vi "CAN_Init - 2013.vi"(0 "设备类型":u32(ring)=4 items=["PCI5121"=1, "PCI9810"=2, "USBCAN1"=3, "USBCAN2"=4, "PCI9820"=5, "CAN232"=6, "PCI5110"=7, "CANLite(mini)"=8, "ISA9620"=9, "ISA5420"=10, "PC104CAN"=11, "CANET"=17, "DNP9810"=13, "USBCAN-E-U"=20, "USBCAN-2E-U"=21], 1 "设备索引":u32(ring) items=["0", "1", "2", "3", "4", "5", "6", "7", "8", "9", "10", "11", "12", "13", "14", "15", ""], 2 "波特率":enum16{"250Kbps", "500Kbps"}(ring)=enum."500Kbps", 3 "CAN路数":u32(ring) items=["0", "1"], 4 "操作类型":enum16{"初始化CAN", "关闭CAN"}(ring), 5 "error in (no error)":errorcluster caption="错误输入（无错误）", 6 "滤波方式":u8(ring)=1 items=["Dual Filter", "Single Filter"], 7 "Accept Code":u32 format="%08x", 8 "IP":string, 9 "port":u32, 10 "工作方式":u8(ring) items=["Normal", "Listen Only"], 11 "Mask Code":u32=4294967295 format="%08x", 12 "PC端-协议类型":enum16{"TCP服务器Server", "TCP客户端Client"}(ring)) -> (14 "CAN 操作结果":bool=TRUE, 19 "error out":errorcluster caption="错误输出")   [LabVIEW 2013]
uses:
  data/ControlCAN.dll
panel:
  in  "VCI_INIT_CONFIG":T1={"AccCode"=0, "AccMask"=4294967295, "Reserved"=0, "Filter"=0, "Timing0"=191, "Timing1"=255, "Mode"=0}
  in  "DeviceType 5":u16(ring)=1 items=["PCI5121"=1, "PCI9810"=2, "USBCAN1"=3, "USBCAN2"=4, "PCI9820"=5, "CAN232"=6, "PCI5110"=7, "CANLite(mini)"=8, "ISA9620"=9, "ISA5420"=10, "PC104CAN"=11, "CANETE"=12, "DNP9810"=13]
  in  "CAN Channel 3":u16(ring) items=["0", "1"]
  in  "DeviceType 4":u16(ring)=1 items=["PCI5121"=1, "PCI9810"=2, "USBCAN1"=3, "USBCAN2"=4, "PCI9820"=5, "CAN232"=6, "PCI5110"=7, "CANLite(mini)"=8, "ISA9620"=9, "ISA5420"=10, "PC104CAN"=11, "CANETE"=12, "DNP9810"=13]
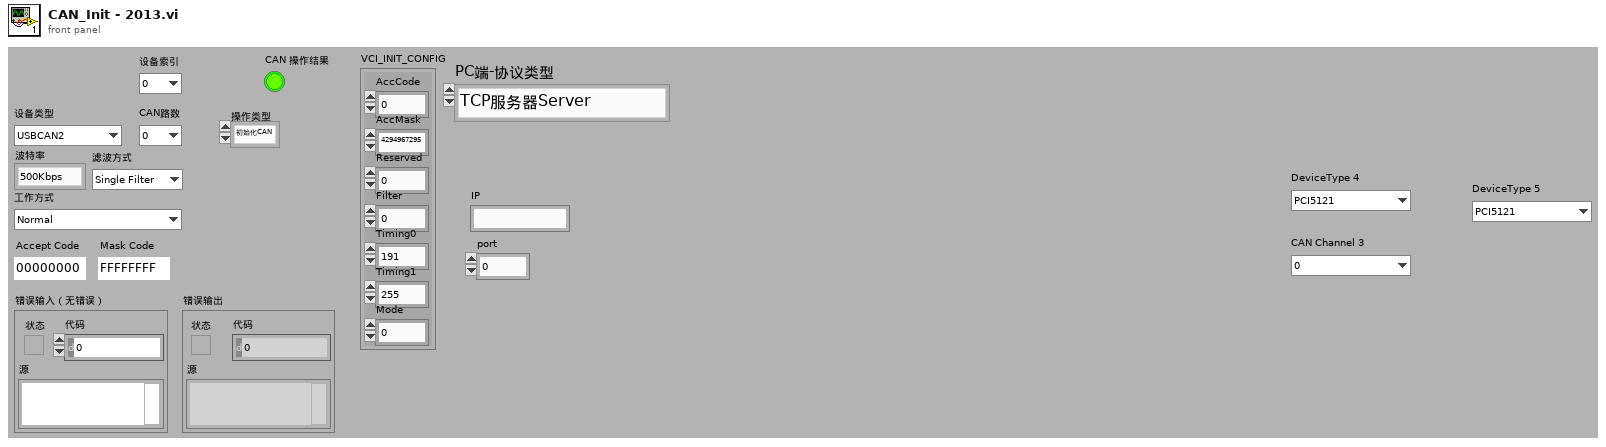
[diagram p1: front panel]
types:
  T1 = cluster{"AccCode":u32, "AccMask":u32, "Reserved":u32, "Filter":u8, "Timing0":u8, "Timing1":u8, "Mode":u8}
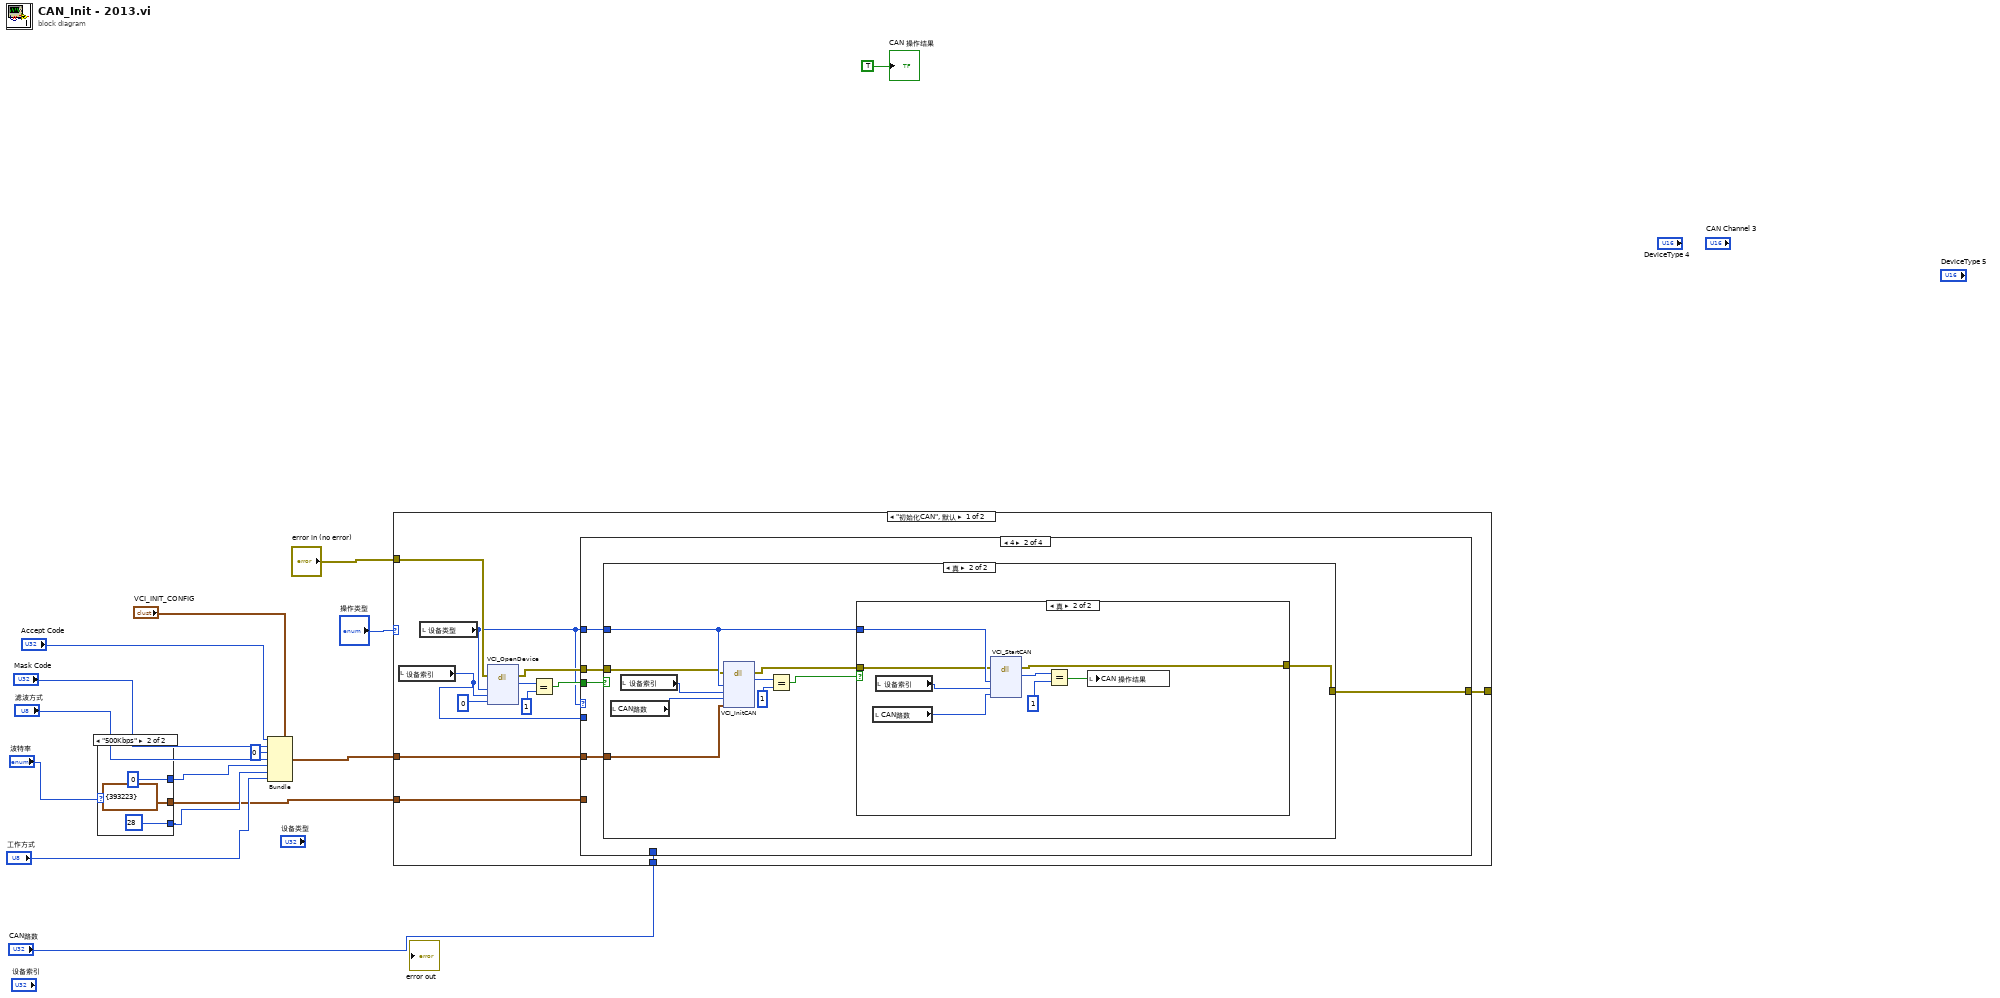
[diagram p0: block diagram]
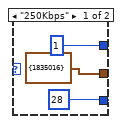
[diagram p2: hidden frame]
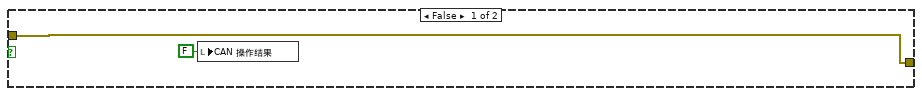
[diagram p4: hidden frame]
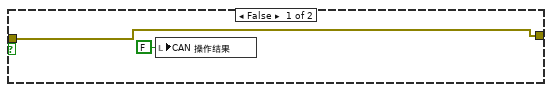
[diagram p5: hidden frame]
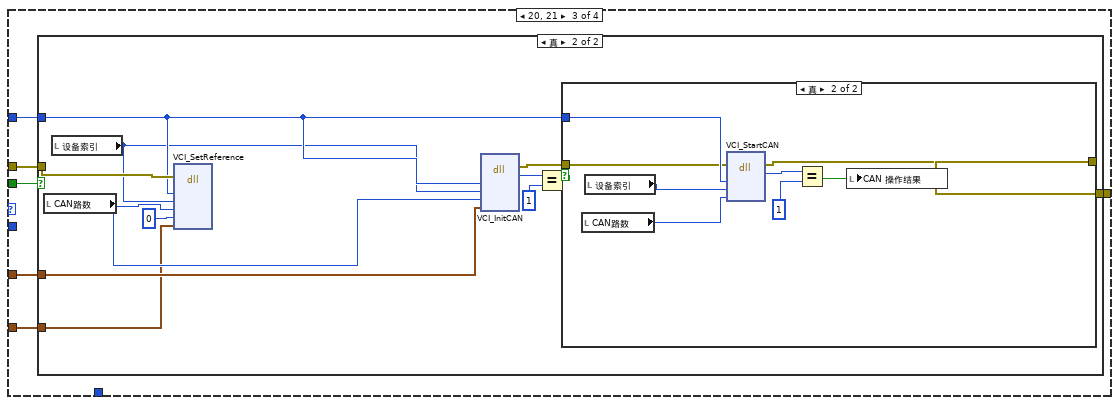
[diagram p6: hidden frame]
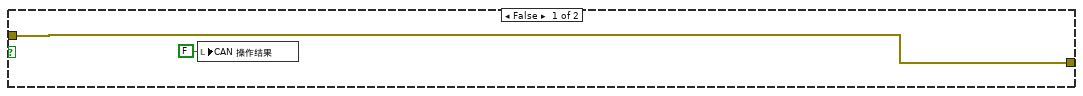
[diagram p7: hidden frame]
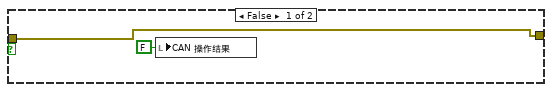
[diagram p8: hidden frame]
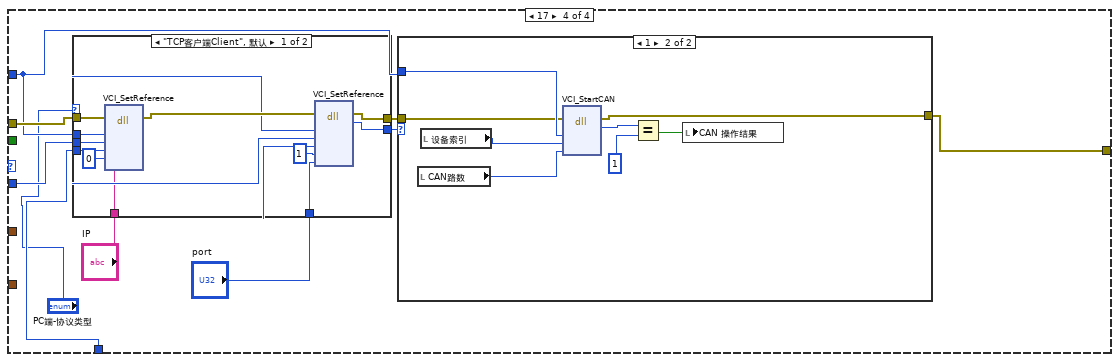
[diagram p9: hidden frame]
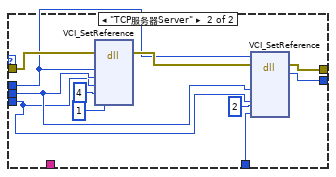
[diagram p10: hidden frame]
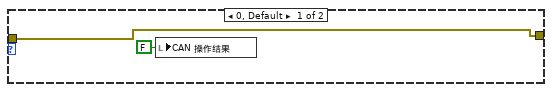
[diagram p11: hidden frame]
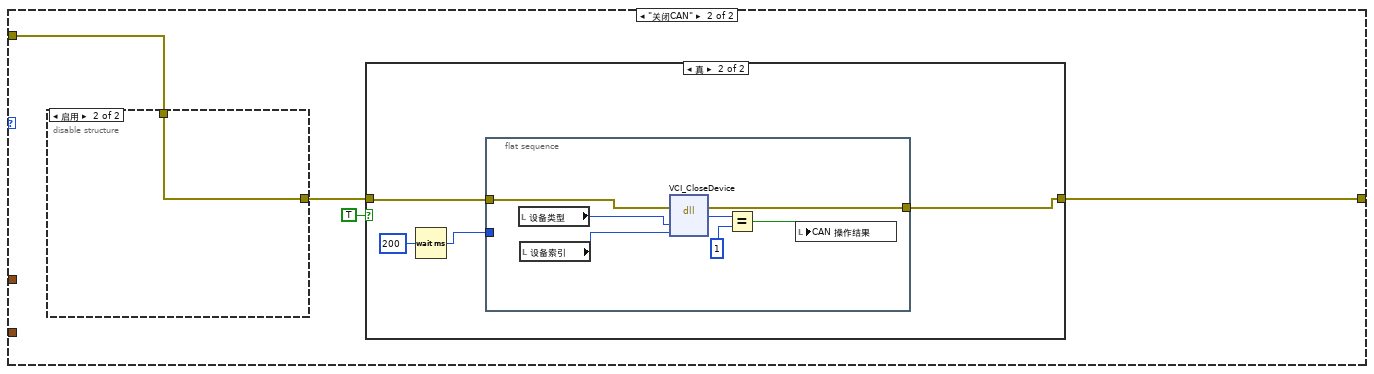
[diagram p12: hidden frame]
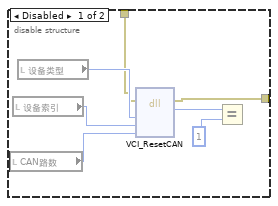
[diagram p13: hidden frame]
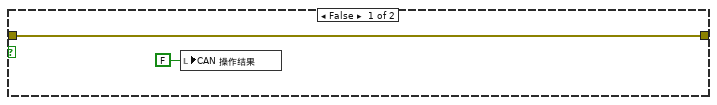
[diagram p14: hidden frame]
diagram:
  n1 = case shown="\"500Kbps\"" "波特率" {
    tunnel: [1 0] -> w14
    tunnel: [28 28] -> w13
    tunnel: [cluster{u32} {1835016} cluster{u32} {393223}] -> w1
    frame "250Kbps" {
    }
    frame "500Kbps" {
    }
  }
  n2 = Bundle(cluster="VCI_INIT_CONFIG", "AccCode"="Accept Code", "AccMask"="Mask Code", "Reserved"=u32 0, "Filter"="滤波方式", "Timing0"=w14, "Timing1"=w13, "Mode"="工作方式") -> (w9:T1)
  n3 = case shown="\"初始化CAN\", 默认" "操作类型" {
    tunnel: w9 -> [w30 _]
    tunnel: "error in (no error)" -> [w29 w137]
    tunnel: [w27 w135] -> _
    tunnel: "CAN路数" -> [w24 _]
    tunnel: w1 -> [w22 _]
    frame "初始化CAN", Default {
      n4 = local read "设备索引"() -> (w25:u32)
      n5 = local read "设备类型"() -> (w23:u32)
      n6 = dll-call lib="PTH1tabs FBluewave New EnergySVN_WorkBMS_Monitor_Bnet01trunkBMS_Monitor_增加二维码dataControlCAN.dll" fn="VCI_OpenDevice"(error in=w29, "DevType"=w23, "DevIndex"=w25, "Reserved"=0) -> (error out=w28:errorcluster, "返回类型"=w32:u32)  [unwired: 3 in, 3 out]
      n7 = Equal?(x=w32, y=u32 1) -> (x = y?=w26:bool)
      n8 = case shown="4" w23 {
        tunnel: w26 -> [_ w39 w67 _]
        tunnel: w23 -> [_ w38 w66 w96]
        tunnel: w30 -> [_ w37 w65 _]
        tunnel: w28 -> [w34 w36 w64 w101]
        tunnel: [w34 w35 w63 w95] -> w27
        tunnel: w25 -> [_ _ _ w100]
        tunnel: w24 -> [_ _ _ w99]
        tunnel: w22 -> [_ _ w62 _]
        frame 0, Default {
        }
        frame 4 {
          n9 = case shown="真" w39 {
            tunnel: w38 -> [_ w46]
            tunnel: w37 -> [_ w45]
            tunnel: w36 -> [w40 w44]
            tunnel: [w40 w42] -> w35
            frame False {
              n10 = local write "CAN 操作结果"(FALSE ("初始化结果")) -> ()
            }
            frame True {
              n11 = local read "CAN路数"() -> (w48:u32)
              n12 = local read "设备索引"() -> (w49:u32)
              n13 = dll-call lib="PTH1tabs FBluewave New EnergySVN_WorkBMS_Monitor_Bnet01trunkBMS_Monitor_增加二维码dataControlCAN.dll" fn="VCI_InitCAN"(error in=w44, "DeviceType"=w46, "DeviceInd"=w49, "CANInd"=w48, "pInitConfig"=w45) -> (error out=w43:errorcluster, "返回类型"=w50:u32)  [unwired: 3 in, 4 out]
              n14 = Equal?(x=w50, y=u32 1) -> (x = y?=w47:bool)
              n15 = case shown="真" w47 {
                tunnel: w46 -> [_ w59]
                tunnel: w43 -> [w52 w55]
                tunnel: [w52 w54] -> w42
                frame False {
                  n16 = local write "CAN 操作结果"(FALSE ("初始化结果")) -> ()
                }
                frame True {
                  n17 = local read "CAN路数"() -> (w57:u32)
                  n18 = local read "设备索引"() -> (w58:u32)
                  n19 = dll-call lib="PTH1tabs FBluewave New EnergySVN_WorkBMS_Monitor_Bnet01trunkBMS_Monitor_增加二维码dataControlCAN.dll" fn="VCI_StartCAN"(error in=w55, "DeviceType"=w59, "DeviceInd"=w58, "CANInd"=w57) -> (error out=w54:errorcluster, "返回类型"=w60:u32)  [unwired: 2 in, 4 out]
                  n20 = Equal?(x=w60, y=u32 1) -> (x = y?=w56:bool)
                  n21 = local write "CAN 操作结果"(w56) -> ()
                }
              }
            }
          }
        }
        frame 20, 21 {
          n22 = case shown="真" w67 {
            tunnel: w66 -> [_ w73]
            tunnel: w65 -> [_ w78]
            tunnel: w64 -> [w68 w75]
            tunnel: [w68 w76] -> w63
            tunnel: w62 -> [_ w70]
            frame False {
              n23 = local write "CAN 操作结果"(FALSE ("初始化结果")) -> ()
            }
            frame True {
              n24 = local read "CAN路数"() -> (w71:u32)
              n25 = local read "设备索引"() -> (w72:u32)
              n26 = dll-call lib="PTH1tabs FBluewave New EnergySVN_WorkBMS_Monitor_Bnet01trunkBMS_Monitor_增加二维码dataControlCAN.dll" fn="VCI_SetReference" label="VCI_SETREF"(error in=w75, "DeviceType"=w73, "DeviceInd"=w72, "CANInd"=w71, "RefType"=u32 0, "pData"=w70) -> ()  [unwired: 4 in, 6 out]
              n27 = dll-call lib="PTH1tabs FBluewave New EnergySVN_WorkBMS_Monitor_Bnet01trunkBMS_Monitor_增加二维码dataControlCAN.dll" fn="VCI_InitCAN"("DeviceType"=w73, "DeviceInd"=w72, "CANInd"=w71, "pInitConfig"=w78) -> (error out=w77:errorcluster, "返回类型"=w80:u32)  [unwired: 4 in, 4 out]
              n28 = Equal?(x=w80, y=u32 1) -> (x = y?=w79:bool)
              n29 = case shown="真" w79 {
                tunnel: w73 -> [_ w89]
                tunnel: w77 -> [w82 w85]
                tunnel: [w82 w84] -> w76
                frame False {
                  n30 = local write "CAN 操作结果"(FALSE ("初始化结果")) -> ()
                }
                frame True {
                  n31 = local read "CAN路数"() -> (w87:u32)
                  n32 = local read "设备索引"() -> (w88:u32)
                  n33 = dll-call lib="PTH1tabs FBluewave New EnergySVN_WorkBMS_Monitor_Bnet01trunkBMS_Monitor_增加二维码dataControlCAN.dll" fn="VCI_StartCAN"(error in=w85, "DeviceType"=w89, "DeviceInd"=w88, "CANInd"=w87) -> (error out=w84:errorcluster, "返回类型"=w90:u32)  [unwired: 2 in, 4 out]
                  n34 = Equal?(x=w90, y=u32 1) -> (x = y?=w86:bool)
                  n35 = local write "CAN 操作结果"(w86) -> ()
                }
              }
            }
          }
        }
        frame 17 {
          n36 = case shown="\"TCP客户端Client\", 默认" "PC端-协议类型" {
            tunnel: w101 -> [w112 w118]
            tunnel: w100 -> [w109 w115]
            tunnel: w99 -> [w108 w114]
            tunnel: [w106 w122] -> w98
            tunnel: [w105 w121] -> w97
            tunnel: w96 -> [w104 w116]
            tunnel: "IP" -> [w103 _]
            tunnel: "port" -> [w102 w120]
            frame "TCP客户端Client", Default {
              n37 = dll-call lib="PTH1tabs FBluewave New EnergySVN_WorkBMS_Monitor_Bnet01trunkBMS_Monitor_增加二维码dataControlCAN.dll" fn="VCI_SetReference" label="VCI_SETREF"(error in=w112, "DeviceType"=w104, "DeviceInd"=w109, "CANInd"=w108, "RefType"=u32 0, "pData"=w103) -> (error out=w110:errorcluster)  [unwired: 4 in, 5 out]
              n38 = dll-call lib="PTH1tabs FBluewave New EnergySVN_WorkBMS_Monitor_Bnet01trunkBMS_Monitor_增加二维码dataControlCAN.dll" fn="VCI_SetReference" label="VCI_SETREF"(error in=w110, "DeviceType"=w104, "DeviceInd"=w109, "CANInd"=w108, "RefType"=u32 1, "pData"=w102) -> (error out=w106:errorcluster, "返回类型"=w105:u32)  [unwired: 4 in, 4 out]
            }
            frame "TCP服务器Server" {
              n39 = dll-call lib="PTH1tabs FBluewave New EnergySVN_WorkBMS_Monitor_Bnet01trunkBMS_Monitor_增加二维码dataControlCAN.dll" fn="VCI_SetReference" label="VCI_SETREF"(error in=w118, "DeviceType"=w116, "DeviceInd"=w115, "CANInd"=w114, "RefType"=u32 4, "pData"=u32 1) -> (error out=w117:errorcluster)  [unwired: 4 in, 5 out]
              n40 = dll-call lib="PTH1tabs FBluewave New EnergySVN_WorkBMS_Monitor_Bnet01trunkBMS_Monitor_增加二维码dataControlCAN.dll" fn="VCI_SetReference" label="VCI_SETREF"(error in=w117, "DeviceType"=w116, "DeviceInd"=w115, "CANInd"=w114, "RefType"=u32 2, "pData"=w120) -> (error out=w122:errorcluster, "返回类型"=w121:u32)  [unwired: 4 in, 4 out]
            }
          }
          n41 = case shown="1" w97 {
            tunnel: w96 -> [_ w131]
            tunnel: w98 -> [w124 w127]
            tunnel: [w124 w126] -> w95
            frame 0, Default {
              n42 = local write "CAN 操作结果"(FALSE ("初始化结果")) -> ()
            }
            frame 1 {
              n43 = local read "CAN路数"() -> (w129:u32)
              n44 = local read "设备索引"() -> (w130:u32)
              n45 = dll-call lib="PTH1tabs FBluewave New EnergySVN_WorkBMS_Monitor_Bnet01trunkBMS_Monitor_增加二维码dataControlCAN.dll" fn="VCI_StartCAN"(error in=w127, "DeviceType"=w131, "DeviceInd"=w130, "CANInd"=w129) -> (error out=w126:errorcluster, "返回类型"=w132:u32)  [unwired: 2 in, 4 out]
              n46 = Equal?(x=w132, y=u32 1) -> (x = y?=w128:bool)
              n47 = local write "CAN 操作结果"(w128) -> ()
            }
          }
        }
      }
    }
    frame "关闭CAN" {
      n48 = disable-structure shown="启用" {
        disable-tunnel: w137 -> [w139 w145]
        disable-tunnel: [w138 w145] -> w136
        frame Disabled {
          n49 = local read "CAN路数"() -> (w140:u32)
          n50 = local read "设备索引"() -> (w141:u32)
          n51 = local read "设备类型"() -> (w142:u32)
          n52 = dll-call lib="PTH1tabs FBluewave New EnergySVN_WorkBMS_Monitor_Bnet01trunkBMS_Monitor_增加二维码dataControlCAN.dll" fn="VCI_ResetCAN"(error in=w139, "DeviceType"=w142, "DeviceInd"=w141, "CANInd"=w140) -> (error out=w138:errorcluster, "返回类型"=w143:u32)  [unwired: 2 in, 4 out]
          n53 = Equal?(x=w143, y=u32 1) -> ()  [unwired: 1 out]
        }
        frame Enabled {
        }
      }
      n54 = case shown="真" TRUE {
        tunnel: w136 -> [w146 w151]
        tunnel: [w146 w150] -> w135
        frame False {
          n55 = local write "CAN 操作结果"(FALSE ("CAN 操作结果")) -> ()
        }
        frame True {
          n56 = Wait (ms)(milliseconds to wait=u32 200 ("等待时间（毫秒）")) -> (millisecond timer value=w148:u32)
          n57 = flat-sequence {
            tunnel: w151 -> [w153]
            tunnel: [w152] -> w150
            tunnel: w148 -> [_]
            frame #0 {
              n58 = local read "设备类型"() -> (w156:u32)
              n59 = local read "设备索引"() -> (w155:u32)
              n60 = dll-call lib="PTH1tabs FBluewave New EnergySVN_WorkBMS_Monitor_Bnet01trunkBMS_Monitor_增加二维码dataControlCAN.dll" fn="VCI_CloseDevice"(error in=w153, "DeviceType"=w156, "DeviceInd"=w155) -> (error out=w152:errorcluster, "返回类型"=w157:u32)  [unwired: 2 in, 3 out]
              n61 = Equal?(x=w157, y=u32 1) -> (x = y?=w154:bool)
              n62 = local write "CAN 操作结果"(w154) -> ()
            }
          }
        }
      }
    }
  }
  "CAN 操作结果" <- TRUE ("CAN 操作结果")
